vi "Problem1.6.vi"() -> ()   [LabVIEW 2019]
panel:
  in  "Deadband":dbl(slide) min=0.0 max=2.0 step=0.25 scale=0.0..2.0
  out "Threshold with Deadband Triggered":bool
  out "Threshold Value Triggered":bool
  out "Slider Value":dbl(knob) scale=0.0..10.0
  in  "Stop":bool
  in  "Threshold":dbl(slide) scale=0.0..10.0
  in  "Slide":dbl(slide) scale=0.0..10.0
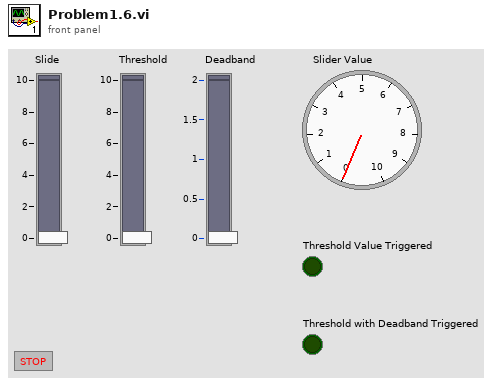
[diagram p1: front panel]
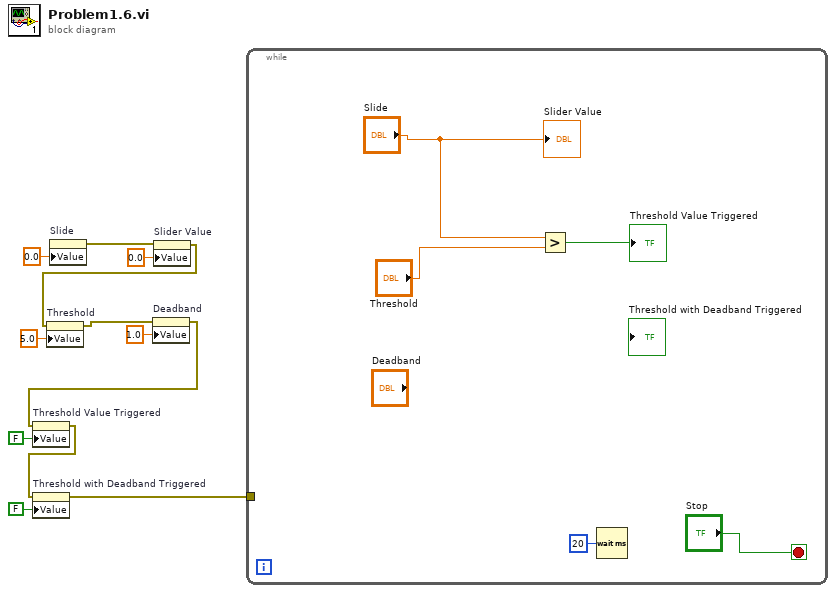
[diagram p0: block diagram]
diagram:
  n1 = property on="Slide" class="Slide (strict)"("Value"=0.0 ("Slide")) -> (error out=w10:errorcluster)  [unwired: 2 in, 1 out]
  n2 = property on="Slider Value" class="Knob (strict)"(error in=w10, "Value"=0.0 ("Slider Value")) -> (error out=w8:errorcluster)  [unwired: 1 in, 1 out]
  n3 = property on="Threshold" class="Slide (strict)"(error in=w8, "Value"=5.0 ("Threshold")) -> (error out=w7:errorcluster)  [unwired: 1 in, 1 out]
  n4 = property on="Deadband" class="Slide (strict)"(error in=w7, "Value"=1.0 ("Deadband")) -> (error out=w4:errorcluster)  [unwired: 1 in, 1 out]
  n5 = property on="Threshold Value Triggered" class="Bool (strict)"(error in=w4, "Value"=FALSE ("Threshold Value Triggered")) -> (error out=w2:errorcluster)  [unwired: 1 in, 1 out]
  n6 = property on="Threshold with Deadband Triggered" class="Bool (strict)"(error in=w2, "Value"=FALSE ("Threshold with Deadband Triggered")) -> (error out=w1:errorcluster)  [unwired: 1 in, 1 out]
  n7 = while {
    tunnel: w1 -> [_]
    stop <- "Stop" stop-if-true
    n8 = Greater?(x="Slide", y="Threshold") -> (0:→"Threshold Value Triggered":bool)
    n9 = Wait (ms)(milliseconds to wait=u32 20) -> ()  [unwired: 1 out]
    "Slider Value" <- "Slide"
  }
